vi "INI Get all value by selection.vi"(7 "File Name":T1, 8 "error in (no error)":errorcluster, 11 "section":string) -> (0 "error out":errorcluster, 1 "transposed array":string[][](array[string]), 2 "Array":string[](array[string]), 3 "key names":string[](array[string]))   [LabVIEW 2021, in "File RW.lvlib"]
doc: "Read all valuse by selection"
uses:
  File RW.lvlib
  FileName.ctl
  <vilib>/Utility/config.llb/Read Key (String).vi
  <vilib>/Utility/config.llb/NI_LVConfig.lvlib
  <userlib>/John_Lib/TopPath/TopPath.lvlib
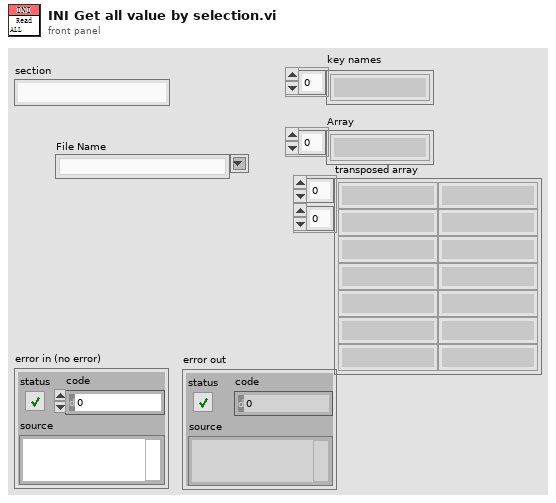
[diagram p1: front panel]
types:
  T1 = typedef "File RW.lvlib/FileName.ctl" = string
  T2 = typedef "NI_LVConfig.lvlib/Config Data RefNum.ctl" = refnum<k1>
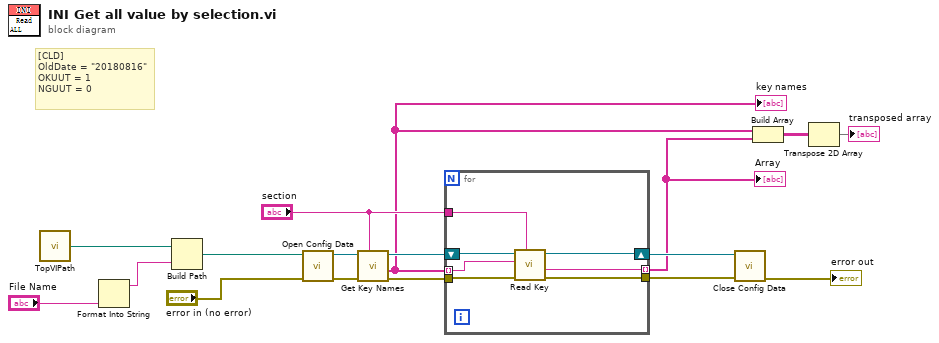
[diagram p0: block diagram]
diagram:
  # "[CLD]\nOldDate = \"20180816\"\nOKUUT = 1    \nNGUUT = 0"
  n1 = call <userlib>:"TopVIPath.vi"() -> ("ConfigFile path"=w1:path)  [unwired: 2 out]
  n2 = Format Into String("File Name") -> (resulting string=w2:string)  [unwired: 3 in, 1 out]
  n3 = Build Path(base path=w1, name or relative path=w2) -> (appended path=w15:path)
  n4 = call <vilib>:"Open Config Data.vi"("error in (no error)"="error in (no error)", "configuration file path"=w15) -> ("error out"=w13:errorcluster, "refnum"=w14:T2)  [unwired: 7 in, 1 out]
  n5 = call <vilib>:"Get Key Names.vi"("section"="section", "error in (no error)"=w13, "refnum"=w14) -> ("error out"=w12:errorcluster, "key names"=w7:string[], "refnum out"=w11:T2)  [unwired: 5 in, 1 out]
  "key names" <- w7
  n6 = for {
    tunnel: w12 -> [w20]
    shift-right: [w21] -> w8
    shift-left: w11 -> [w22]
    tunnel: w7 -> [w24] mode=indexing
    tunnel: "section" -> [w23]
    tunnel: [w19] -> w9
    tunnel: [w18] -> w6 mode=indexing
    n7 = call-poly <vilib>:"Read Key.vi"("section"=w23, "error in (no error)"=w20, "key"=w24, "refnum"=w22) -> ("error out"=w19:errorcluster, "value"=w18:string, "refnum out"=w21:T2)  [unwired: 4 in, 1 out]
  }
  "Array" <- w6
  n8 = call <vilib>:"Close Config Data.vi"("error in (no error)"=w9, "refnum"=w8) -> ("error out"=→"error out":errorcluster)  [unwired: 8 in, 1 out]
  n9 = Build Array(w7, w6) -> (w5:string[][])
  n10 = Transpose 2D Array(2D array=w5) -> (transposed array=→"transposed array":string[][])
